vi "Wave2D_Init Data_BC.vi"(6 "delta y":dbl, 8 "kq":dbl, 9 "delta x":dbl, 10 "kp":dbl, 11 "Boundary Condition":cluster{"type":T2, "Value":dbl[][]}[](array[cluster]) {"type" items=["Dirichlet", "Neumann"]}) -> (2 "Corner":T1, 3 "BC":T3 {"End Y"."type" items=["Dirichlet", "Neumann"]; "Start Y"."type" items=["Dirichlet", "Neumann"]; "End X"."type" items=["Dirichlet", "Neumann"]; "Start X"."type" items=["Dirichlet", "Neumann"]})   [LabVIEW 2017, in "NI_PDE.lvlib"]
uses:
  <vilib>/gmath/NI_PDE.lvlib
  <vilib>/gmath/pde.llb/Common/PDE_BC Type.ctl
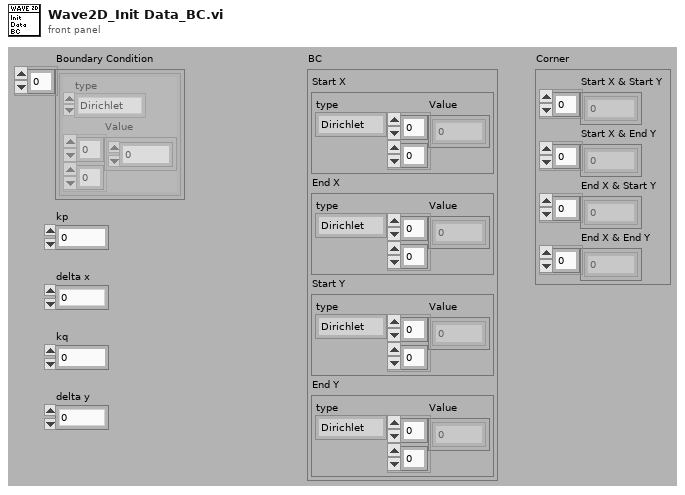
[diagram p1: front panel]
types:
  T1 = cluster{"Start X & Start Y":dbl[], "Start X & End Y":dbl[], "End X & Start Y":dbl[], "End X & End Y":dbl[]}
  T2 = typedef "NI_PDE.lvlib/PDE_BC Type.ctl" = i32
  T3 = cluster{"Start X":cluster{"type":T2, "Value":dbl[][]}, "End X":cluster{"type":T2, "Value":dbl[][]}, "Start Y":cluster{"type":T2, "Value":dbl[][]}, "End Y":cluster{"type":T2, "Value":dbl[][]}}
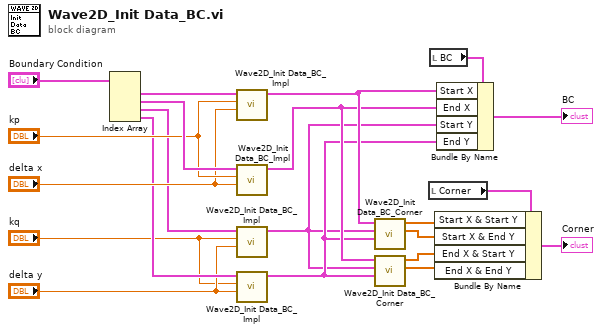
[diagram p0: block diagram]
diagram:
  n1 = Index Array(array="Boundary Condition") -> (element #1=w20:cluster{"type":T2, "Value":dbl[][]}, element #2=w19:cluster{"type":T2, "Value":dbl[][]}, element #3=w14:cluster{"type":T2, "Value":dbl[][]}, element #4=w13:cluster{"type":T2, "Value":dbl[][]})  [unwired: 4 in]
  n2 = call <vilib>:"Wave2D_Init Data_BC_Impl.vi"("delta"="delta x", "k"="kp", "Boundary Condition"=w20) -> ("BC"=w10:cluster{"type":T2, "Value":dbl[][]})  [unwired: 8 out]
  n3 = call <vilib>:"Wave2D_Init Data_BC_Impl.vi"("delta"="delta x", "k"="kp", "Boundary Condition"=w19) -> ("BC"=w9:cluster{"type":T2, "Value":dbl[][]})  [unwired: 8 out]
  n4 = call <vilib>:"Wave2D_Init Data_BC_Impl.vi"("delta"="delta y", "k"="kq", "Boundary Condition"=w14) -> ("BC"=w7:cluster{"type":T2, "Value":dbl[][]})  [unwired: 8 out]
  n5 = call <vilib>:"Wave2D_Init Data_BC_Impl.vi"("delta"="delta y", "k"="kq", "Boundary Condition"=w13) -> ("BC"=w8:cluster{"type":T2, "Value":dbl[][]})  [unwired: 8 out]
  n6 = call <vilib>:"Wave2D_Init Data_BC_Corner.vi"("End Y"=w8, "Start Y"=w7, "X"=w10) -> ("X & End Y"=w4:dbl[], "X & Start Y"=w5:dbl[])  [unwired: 7 out]
  n7 = call <vilib>:"Wave2D_Init Data_BC_Corner.vi"("End Y"=w8, "Start Y"=w7, "X"=w9) -> ("X & End Y"=w2:dbl[], "X & Start Y"=w3:dbl[])  [unwired: 7 out]
  n8 = local read "Corner"() -> (w6:T1)
  n9 = local read "BC"() -> (w16:T3)
  n10 = Bundle By Name(cluster=w6, "Start X & Start Y"=w5, "Start X & End Y"=w4, "End X & Start Y"=w3, "End X & End Y"=w2) -> (→"Corner":T1)
  n11 = Bundle By Name(cluster=w16, "Start X"=w10, "End X"=w9, "Start Y"=w7, "End Y"=w8) -> (→"BC":T3)
